vi "quadrant_check.vi"(9 "Sektor":T1, 10 "y":dbl, 11 "x":dbl) -> (3 "Quadrant OK":bool)   [LabVIEW 2019, in "Kreisquadrant.lvclass"]
uses:
  Kreisquadrant/Kreisquadrant.lvclass
  Quadrant.ctl
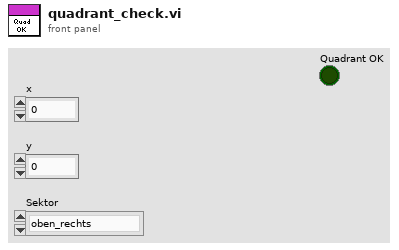
[diagram p1: front panel]
types:
  T1 = typedef "Quadrant.ctl" = enum16{"oben_rechts", "oben_links", "unten_links", "unten_rechts"}
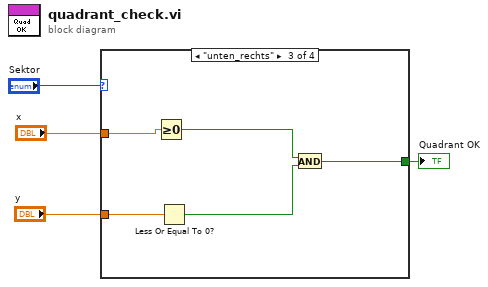
[diagram p0: block diagram]
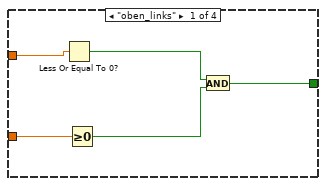
[diagram p2: hidden frame]
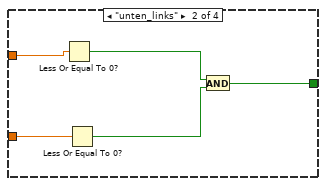
[diagram p3: hidden frame]
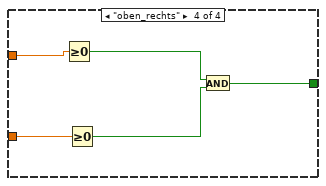
[diagram p4: hidden frame]
diagram:
  n1 = case shown="\"unten_rechts\"" "Sektor" {
    tunnel: [w7 w12 w17 w22] -> w3
    tunnel: "x" -> [w6 w11 w16 w21]
    tunnel: "y" -> [w5 w10 w15 w20]
    frame "oben_links" {
      n2 = Less Or Equal To 0?(x=w6) -> (x <= 0?=w9:bool)
      n3 = Greater Or Equal To 0?(x=w5) -> (x >= 0?=w8:bool)
      n4 = And(x=w9, y=w8) -> (x .and. y?=w7:bool)
    }
    frame "unten_links" {
      n5 = Less Or Equal To 0?(x=w11) -> (x <= 0?=w14:bool)
      n6 = Less Or Equal To 0?(x=w10) -> (x <= 0?=w13:bool)
      n7 = And(x=w14, y=w13) -> (x .and. y?=w12:bool)
    }
    frame "unten_rechts" {
      n8 = Greater Or Equal To 0?(x=w16) -> (x >= 0?=w19:bool)
      n9 = Less Or Equal To 0?(x=w15) -> (x <= 0?=w18:bool)
      n10 = And(x=w19, y=w18) -> (x .and. y?=w17:bool)
    }
    frame "oben_rechts" {
      n11 = Greater Or Equal To 0?(x=w21) -> (x >= 0?=w24:bool)
      n12 = Greater Or Equal To 0?(x=w20) -> (x >= 0?=w23:bool)
      n13 = And(x=w24, y=w23) -> (x .and. y?=w22:bool)
    }
  }
  "Quadrant OK" <- w3
